vi "Read Overlay Positions.vi"(8 "error in (no error)":errorcluster, 11 "Analyze Results Distanz in":refnum<class "Analyze Results Distanz.lvclass">) -> (0 "error out":errorcluster, 2 "Overlay Positions":cluster{"x":i16, "y":i16}[](array[cluster]), 3 "Analyze Results Distanz out":refnum<class "Analyze Results Distanz.lvclass">)   [LabVIEW 2014, in "Analyze Results Distanz.lvclass"]
uses:
  Analyze Results Distanz.lvclass
  Analyze Results Distanz.lvclass/Analyze Results Distanz.ctl
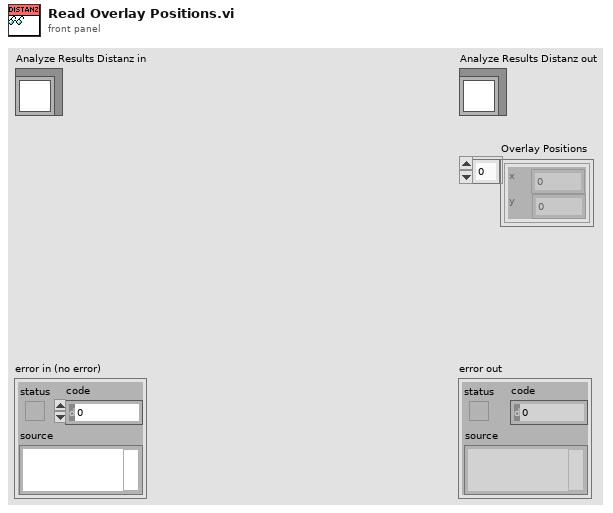
[diagram p1: front panel]
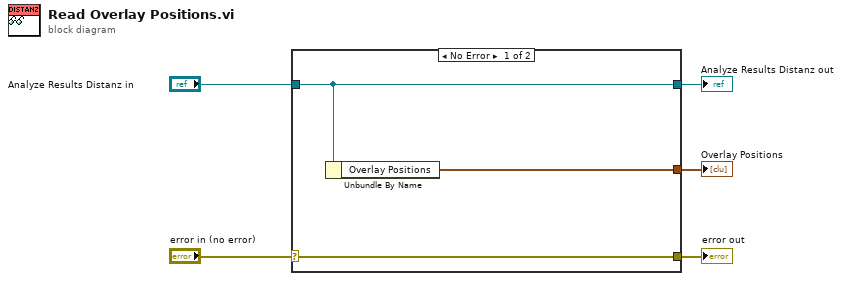
[diagram p0: block diagram]
diagram:
  n1 = case shown="No Error" "error in (no error)" {
    selector: "error in (no error)" -> [w8 w9]
    tunnel: [w8 w9] -> w4
    tunnel: [w7 w10] -> w2
    tunnel: "Analyze Results Distanz in" -> [w7 w10]
    tunnel: [w6 _] -> w1
    frame No Error {
      n2 = Unbundle By Name(w7) -> ("Overlay Positions"=w6:cluster{"x":i16, "y":i16}[])
    }
    frame Error {
    }
  }
  "error out" <- w4
  "Analyze Results Distanz out" <- w2
  "Overlay Positions" <- w1
